vi "TCP Loop - Client as Consumer.vi"(6 "params":T2={"Open timeout(ms)"=50, "Trans timeout(ms)"=200, "idle time(ms)"=100}, 8 "error in (no error)":errorcluster, 9 "port":u16=4008, 10 "ip address":string="127.0.0.1", 11 "DataQueue":refnum<queue>) -> (0 "error out":errorcluster)   [LabVIEW 2017]
doc: "TCP transmission loop acting as the client. It connects to ip address:port and dequeues strings from DataQueue, sending each one over the connection. params sets the open timeout, the transmission timeout and the idle time in ms."
panel:
  out "State":T1(ring)
  out "idle time(ms)":i32
  out "current time":timestamp
  out "datalength":i32
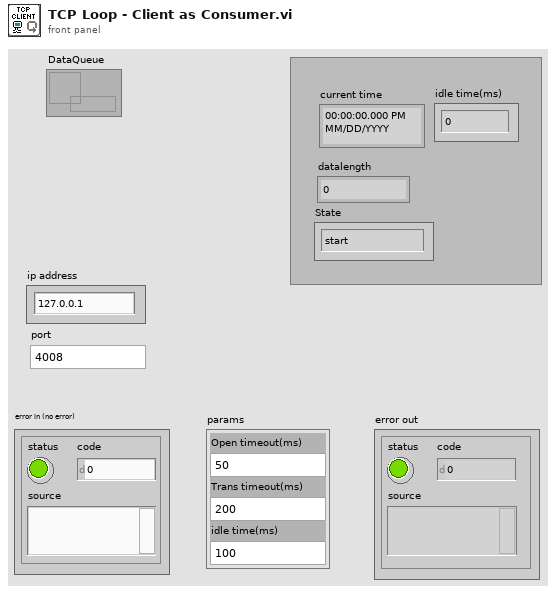
[diagram p1: front panel]
types:
  T1 = enum16{"start", "Connect", "Work", "Close", "Stop loop"}
  T2 = cluster{"Open timeout(ms)":i32, "Trans timeout(ms)":i32, "idle time(ms)":i32}
  T3 = enum16{"Standard", "Buffered", "CRLF", "Immediate"}
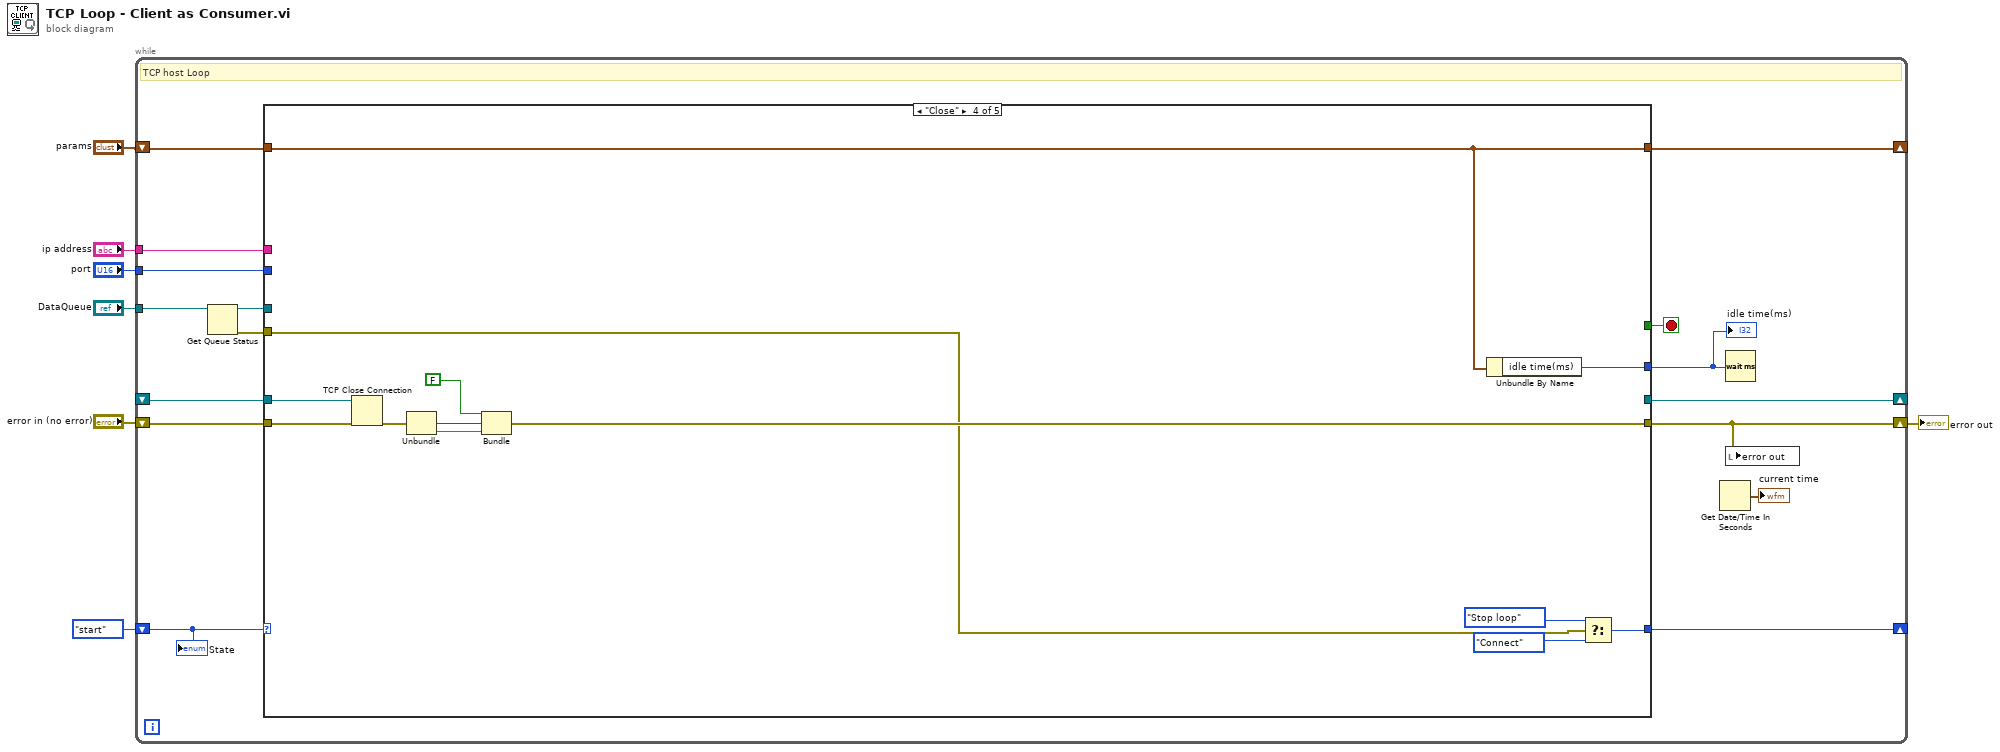
[diagram p0: block diagram]
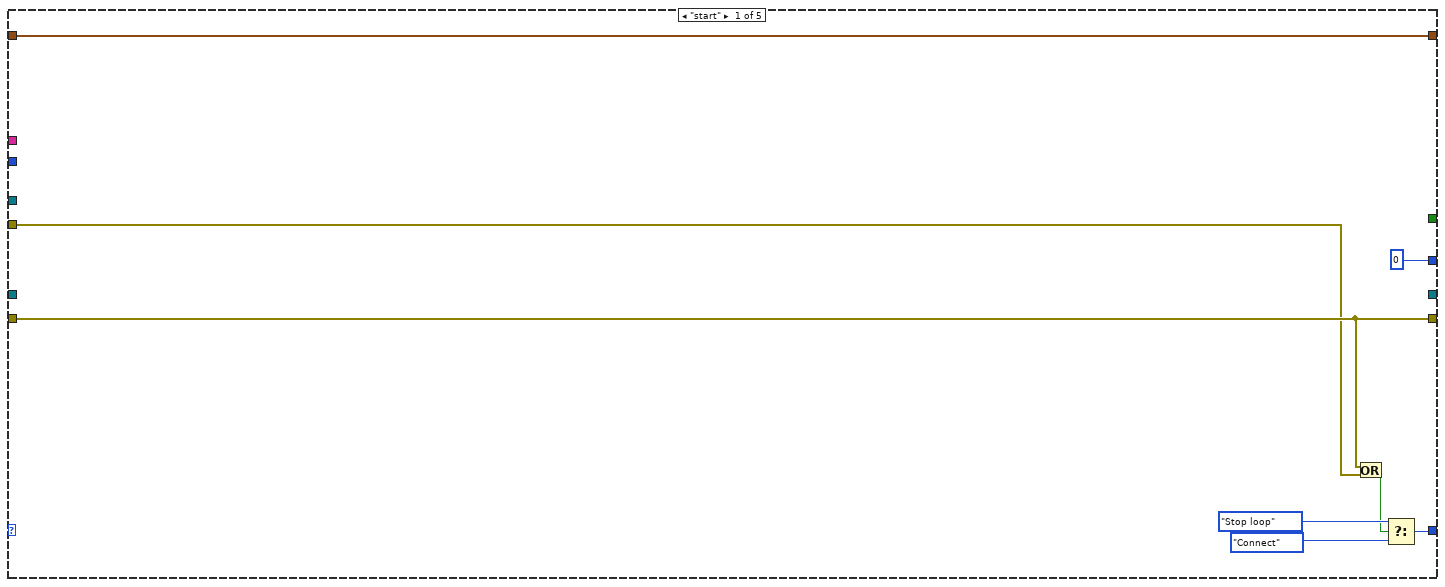
[diagram p2: hidden frame]
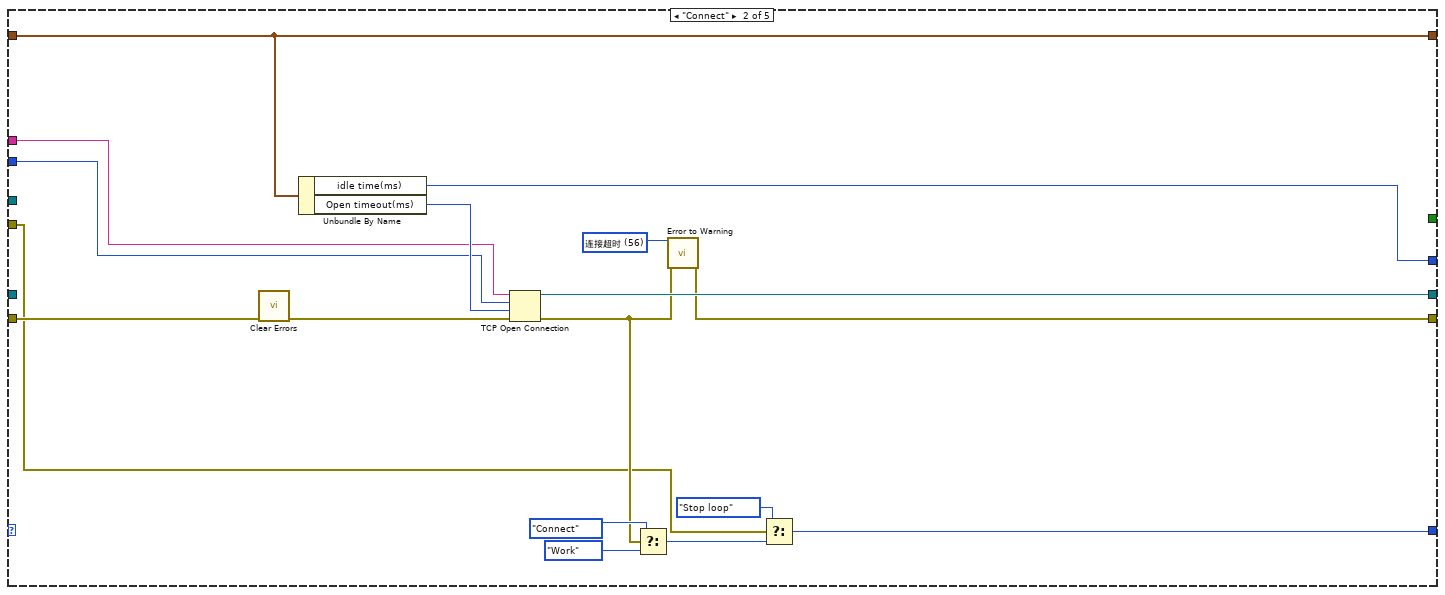
[diagram p3: hidden frame]
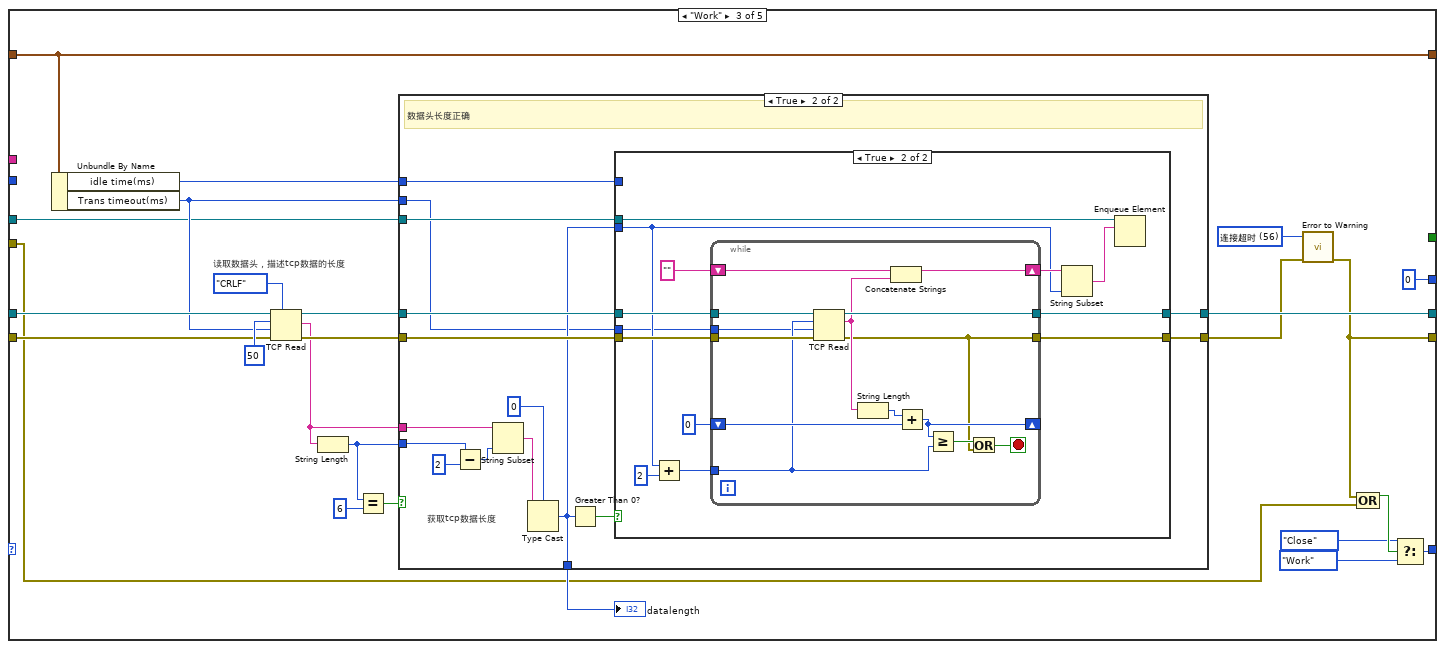
[diagram p4: hidden frame]
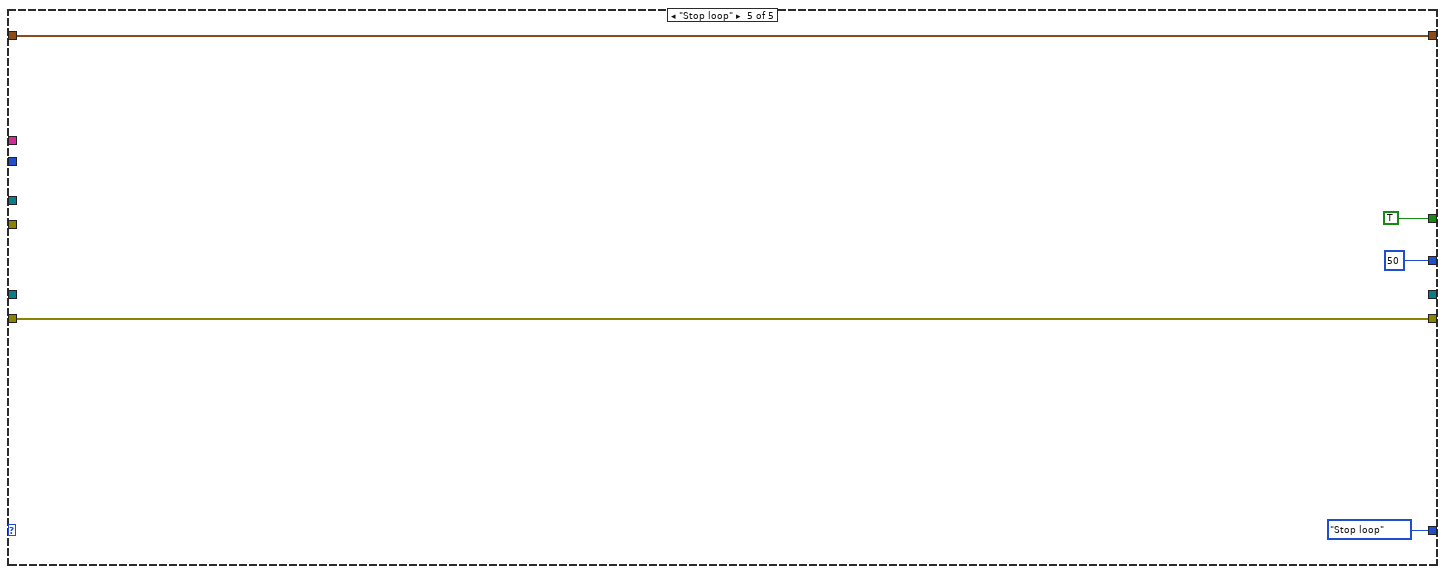
[diagram p7: hidden frame]
diagram:
  n1 = while {
    shift-right: [w17] -> _
    shift-left: T1."start" -> [w16]
    shift-right: [w23] -> _
    shift-left: _ -> [w22]
    shift-right: [w13] -> _
    shift-left: "params" -> [w18]
    shift-right: [w8] -> w5
    shift-left: "error in (no error)" -> [w20]
    tunnel: "DataQueue" -> [w15]
    tunnel: "ip address" -> [w11]
    tunnel: "port" -> [w10]
    stop <- w21 stop-if-true
    # "TCP host Loop"
    n2 = Get Queue Status(queue=w15) -> (queue out=w14:refnum<queue>, error out=w12:errorcluster)  [unwired: 2 in, 6 out]
    n3 = case shown="\"Close\"" w16 {
      tunnel: [_ w48 w66 _ _] -> w23
      tunnel: [w29 w41 w70 w127 T1."Stop loop"] -> w17
      tunnel: w22 -> [_ _ w72 w131 _]
      tunnel: [_ _ _ _ TRUE] -> w21
      tunnel: w20 -> [w26 w45 w71 w130 w136]
      tunnel: [w26 w47 w50 w123 w136] -> w8
      tunnel: [0 w37 0 ("idle time(ms)") w126 50] -> w19
      tunnel: w18 -> [w25 w35 w54 w121 w133]
      tunnel: w14 -> [_ _ w55 _ _]
      tunnel: [w25 w35 w54 w121 w133] -> w13
      tunnel: w12 -> [w24 w34 w53 w120 _]
      tunnel: w11 -> [_ w33 _ _ _]
      tunnel: w10 -> [_ w32 _ _ _]
      frame "start" {
        n4 = Or(x=w26, y=w24) -> (x .or. y?=w27:bool)
        n5 = Select(t=T1."Stop loop", s=w27, f=T1."Connect") -> (s? t:f=w29:T1)
      }
      frame "Connect" {
        w46 = 56 items=["无错误", "参数错误", "内存已满", "超出区域", "文件结束", "文件已打开", "一般文件IO错误", "未找到文件", "文件权限错误", "磁盘已满", "路径副本", "打开过多文件", "未启用", "未找到资源文件", "无法添加资源", "未找到资源", "未找到图像", "图像内存错误", "画笔不存在", "配置错误类型", "配置未找到解析段", "配置解析错误", "配置内存错误", "错误外部代码格式", "错误外部代码偏移量", "外部代码不存在", "空窗口", "销毁窗口错误", "空菜单", "打印已中止", "错误打印记录", "打印驱动程序错误", "打印时窗口错误", "打印时内存错误", "打印对话框错误", "一般打印错误", "无效设备引用句柄", "设备未找到", "设备参数错误", "设备单位错误", "无法打开设备", "设备调用已中止", "一般错误", "用户已取消", "对象ID过低", "对象ID过高", "对象不在堆中", "未知的堆", "错误DefProc ID", "DefProc不在表格中", "范围外信息", "空方法", "未知信息", "不支持管理器调用", "错误地址", "连接过程中", "连接超时", "连接过程中", "不支持网络属性", "网络错误", "正在使用的地址", "系统缺少内存", "连接已中止", "连接已拒绝", "连接未建立", "连接已建立", "连接已关闭", "初始化错误（交互应用程序管理器）", "错误事件发生", "等待无约束事件发生处理程序", "事件发生队列溢出", "错误路径", "未发出信号量", "未识别类型（交互应用程序管理器）"] ("2nd Error to Convert")
        n6 = call <vilib>:"Clear Errors.vi"("error in (no error)"=w45) -> ("error out"=w38:errorcluster)  [unwired: 5 in, 1 out]
        n7 = Unbundle By Name(w35) -> ("idle time(ms)"=w37:i32, "Open timeout(ms)"=w44:i32)
        n8 = TCP Open Connection(address=w33, remote port or service name=w32, timeout ms (60000)=w44, error in (no error)=w38) -> (connection ID=w48:refnum<k5>, error out=w36:errorcluster)  [unwired: 1 in]
        n9 = Select(t=T1."Connect", s=w36, f=T1."Work") -> (s? t:f=w39:T1)
        n10 = call <vilib>:"Error to Warning.vi"("1st Error to Convert"=w46, "error in (no error)"=w36) -> ("warning out"=w47:errorcluster)  [unwired: 13 in]
        n11 = Select(t=T1."Stop loop", s=w34, f=w39) -> (s? t:f=w41:T1)
      }
      frame "Work" {
        w52 = 56 items=["无错误", "参数错误", "内存已满", "超出区域", "文件结束", "文件已打开", "一般文件IO错误", "未找到文件", "文件权限错误", "磁盘已满", "路径副本", "打开过多文件", "未启用", "未找到资源文件", "无法添加资源", "未找到资源", "未找到图像", "图像内存错误", "画笔不存在", "配置错误类型", "配置未找到解析段", "配置解析错误", "配置内存错误", "错误外部代码格式", "错误外部代码偏移量", "外部代码不存在", "空窗口", "销毁窗口错误", "空菜单", "打印已中止", "错误打印记录", "打印驱动程序错误", "打印时窗口错误", "打印时内存错误", "打印对话框错误", "一般打印错误", "无效设备引用句柄", "设备未找到", "设备参数错误", "设备单位错误", "无法打开设备", "设备调用已中止", "一般错误", "用户已取消", "对象ID过低", "对象ID过高", "对象不在堆中", "未知的堆", "错误DefProc ID", "DefProc不在表格中", "范围外信息", "空方法", "未知信息", "不支持管理器调用", "错误地址", "连接过程中", "连接超时", "连接过程中", "不支持网络属性", "网络错误", "正在使用的地址", "系统缺少内存", "连接已中止", "连接已拒绝", "连接未建立", "连接已建立", "连接已关闭", "初始化错误（交互应用程序管理器）", "错误事件发生", "等待无约束事件发生处理程序", "事件发生队列溢出", "错误路径", "未发出信号量", "未识别类型（交互应用程序管理器）"] ("2nd Error to Convert")
        # "读取数据头，描述tcp数据的长度"
        n12 = Unbundle By Name(w54) -> ("idle time(ms)"=w56:i32, "Trans timeout(ms)"=w59:i32)
        n13 = TCP Read(connection ID=w72, bytes to read=50, error in (no error)=w71, 7:T3."CRLF" ("mode (standard)"), 9:w59) -> (connection ID out=w67:refnum<k5>, data out=w64:string, error out=w68:errorcluster)
        n14 = String Length(string=w64) -> (length=w63:i32)
        n15 = Equal?(x=w63, y=6) -> (x = y?=w61:bool)
        n16 = case shown="True" w61 {
          tunnel: w68 -> [w75 w90]
          tunnel: [w75 w89] -> w51
          tunnel: w67 -> [w74 w88]
          tunnel: [w74 w87] -> w66
          tunnel: w55 -> [_ w85]
          tunnel: w64 -> [_ w82]
          tunnel: w63 -> [_ w79]
          tunnel: [_ w78] -> w60
          tunnel: w59 -> [_ w77]
          tunnel: w56 -> [_ w76]
          frame False {
            # "并非数据头"
          }
          frame True {
            # "获取tcp数据长度"
            # "数据头长度正确"
            n17 = Subtract(x=w79, y=2) -> (x-y=w83:i32)
            n18 = String Subset(string=w82, length (rest)=w83) -> (substring=w81:string)  [unwired: 1 in]
            n19 = Type Cast(type=0 ("y"), x=w81) -> (*(type *) &x=w78:i32)
            n20 = Greater Than 0?(x=w78) -> (x > 0?=w86:bool)
            n21 = case shown="True" w86 {
              tunnel: w90 -> [w91 w105]
              tunnel: [w91 w104] -> w89
              tunnel: w88 -> [w92 w103]
              tunnel: [w92 w102] -> w87
              tunnel: w85 -> [_ w101]
              tunnel: w78 -> [_ w94]
              tunnel: w77 -> [_ w93]
              tunnel: w76 -> [_ _]
              frame False {
              }
              frame True {
                n22 = Add(x=w94, y=2) -> (x+y=w99:i32)
                n23 = while {
                  tunnel: w105 -> [w119]
                  tunnel: [w107] -> w104
                  tunnel: w103 -> [w118]
                  tunnel: [w117] -> w102
                  tunnel: w99 -> [w111]
                  shift-right: [w110] -> _
                  shift-left: 0 ("y") -> [w112]
                  shift-right: [w116] -> w96
                  shift-left: "" -> [w115]
                  tunnel: w93 -> [w106]
                  stop <- w108 stop-if-true
                  n24 = TCP Read(connection ID=w118, bytes to read=w111, error in (no error)=w119, 9:w106) -> (connection ID out=w117:refnum<k5>, data out=w114:string, error out=w107:errorcluster)  [unwired: 1 in]
                  n25 = String Length(string=w114) -> (length=w113:i32)
                  n26 = Concatenate Strings(w115, w114) -> (w116:string)
                  n27 = Add(x=w113, y=w112) -> (x+y=w110:i32)
                  n28 = Greater Or Equal?(x=w110, y=w111) -> (x >= y?=w109:bool)
                  n29 = Or(x=w109, y=w107) -> (x .or. y?=w108:bool)
                }
                n30 = String Subset(string=w96, length (rest)=w94) -> (substring=w95:string)  [unwired: 1 in]
                n31 = Enqueue Element(queue=w101, element=w95) -> ()  [unwired: 2 in, 3 out]
              }
            }
          }
        }
        "datalength" <- w60
        n32 = call <vilib>:"Error to Warning.vi"("1st Error to Convert"=w52, "error in (no error)"=w51) -> ("warning out"=w50:errorcluster)  [unwired: 13 in]
        n33 = Compound Arithmetic op=OR(w50, w53) -> (w69:bool)
        n34 = Select(t=T1."Close", s=w69, f=T1."Work") -> (s? t:f=w70:T1)
      }
      frame "Close" {
        n35 = TCP Close Connection(connection ID=w131, error in (no error)=w130) -> (error out=w132:errorcluster)  [unwired: 1 in, 1 out]
        n36 = Unbundle(w132) -> ("code"=w125:i32, "source"=w124:string)  [unwired: 1 out]
        n37 = Bundle(FALSE, "code"=w125, "source"=w124) -> (w123:cluster{bool, "code":i32, "source":string})  [unwired: 1 in]
        n38 = Unbundle By Name(w121) -> ("idle time(ms)"=w126:i32)
        n39 = Select(t=T1."Stop loop", s=w120, f=T1."Connect") -> (s? t:f=w127:T1)
      }
      frame "Stop loop" {
      }
    }
    "idle time(ms)" <- w19
    n40 = Get Date/Time In Seconds() -> (seconds since 1Jan1904=→"current time":timestamp)
    n41 = Wait (ms)(milliseconds to wait=w19) -> ()  [unwired: 1 out]
    n42 = local write "error out"(w8) -> ()
    "State" <- w16
  }
  "error out" <- w5
